vi "MeasureFastIV.vi"(0 ".NET Refnum in":refnum<k24>, 1 ".NET Refnum":refnum<k24>, 2 "Junction Name":string, 7 "appended path":path, 12 "new file path (Not A Path if cancelled)":path, 13 "UiDefinition":T1, 14 "Function":string) -> (15 "error out":errorcluster)   [LabVIEW 2020]
uses:
  D:/LabviewDXFViewer/LabviewDXFViewer/bin/Release/LabviewDXFViewer.exe
  LabviewDXFViewer/bin/Release/LabviewDXFViewer.exe
  UIReferences.ctl
  <vilib>/Analysis/6fits.llb/Curve Fitting Criteria.ctl
  <vilib>/Utility/file.llb/Write Delimited Spreadsheet (DBL).vi
  <vilib>/Utility/file.llb/Write Delimited Spreadsheet (string).vi
  <vilib>/Analysis/NI_AALPro.lvlib
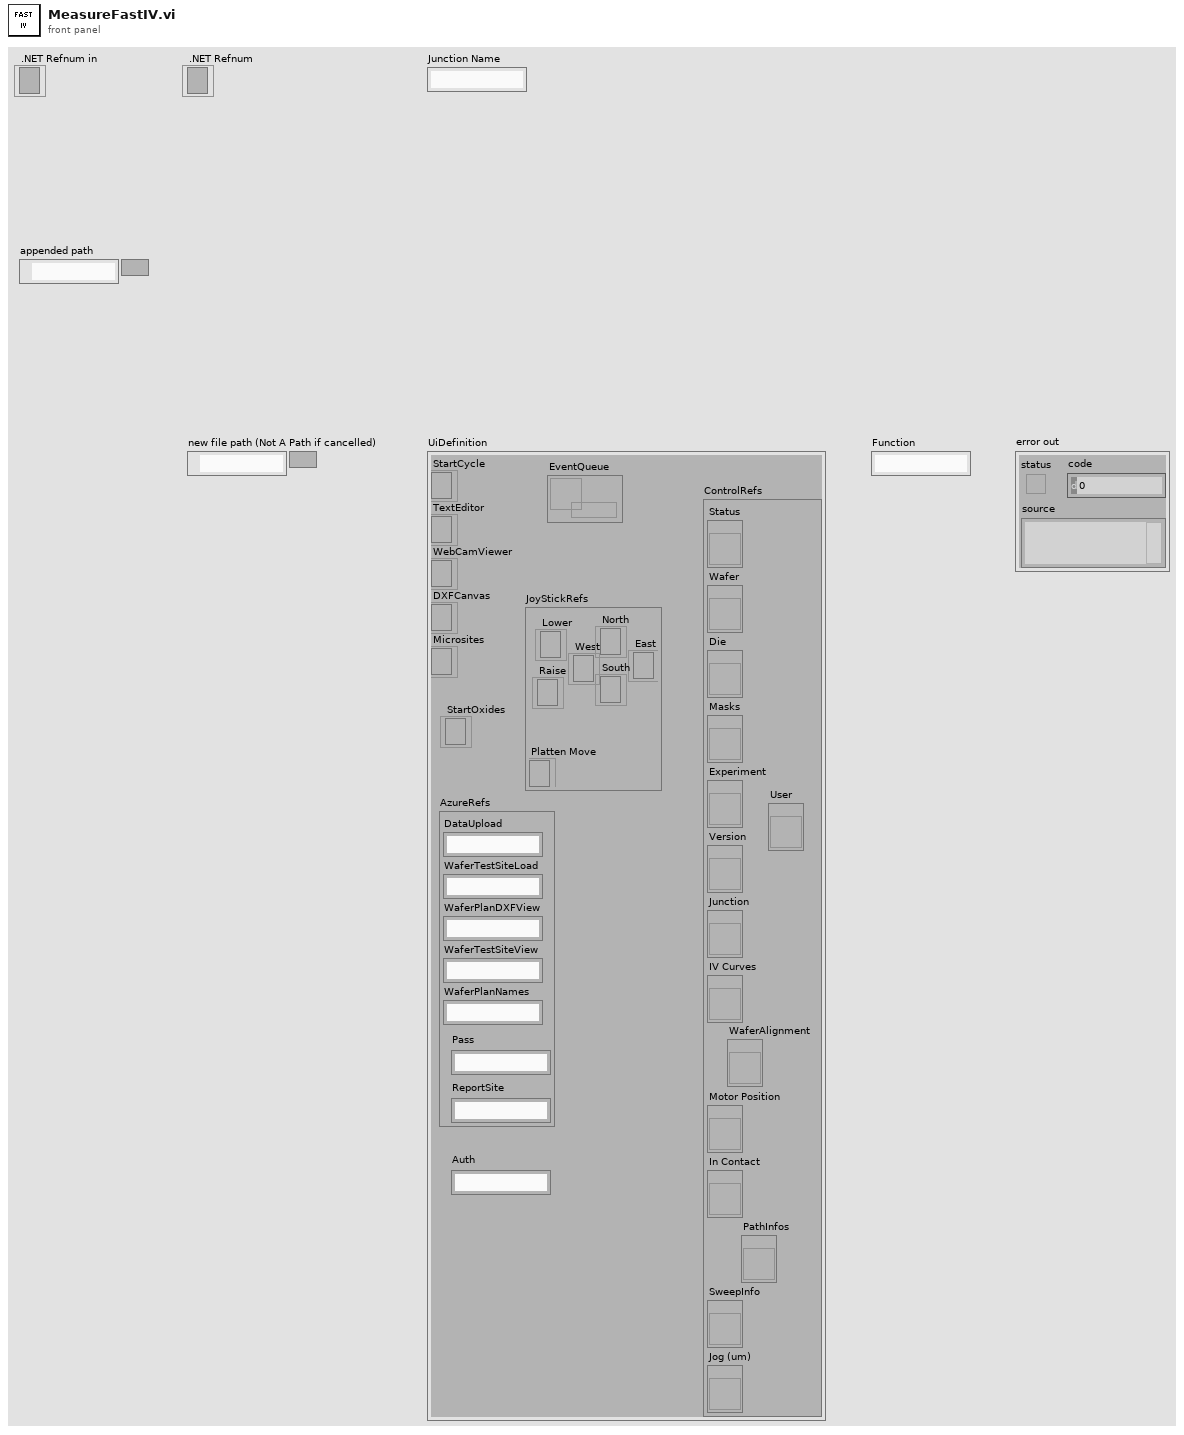
[diagram p1: front panel]
types:
  T1 = typedef "UIReferences.ctl" = cluster{"StartCycle":refnum<k24>, "TextEditor":refnum<k24>, "WebCamViewer":refnum<k24>, "DXFCanvas":refnum<k24>, "Microsites":refnum<k24>, "JoyStickRefs":cluster{"North":refnum<k24>, "Lower":refnum<k24>, "Raise":refnum<k24>, "Platten Move":refnum<k24>, "West":refnum<k24>, "East":refnum<k24>, "South":refnum<k24>}, "AzureRefs":cluster{"DataUpload":string, "WaferTestSiteLoad":string, "WaferPlanDXFView":string, "WaferTestSiteView":string, "WaferPlanNames":string, "Pass":string, "ReportSite":string}, "ControlRefs":cluster{"Status":refnum<vi>, "Wafer":refnum<vi>, "Die":refnum<vi>, "Masks":refnum<vi>, "Experiment":refnum<vi>, "Version":refnum<vi>, "Junction":refnum<vi>, "IV Curves":refnum<vi>, "Motor Position":refnum<vi>, "In Contact":refnum<vi>, "SweepInfo":refnum<vi>, "Jog (um)":refnum<vi>, "PathInfos":refnum<vi>, "User":refnum<vi>, "WaferAlignment":refnum<vi>}, "EventQueue":refnum<queue>, "StartOxides":refnum<k24>, "Auth":string}
  T2 = typedef "NI_AALPro.lvlib/Curve Fitting Criteria.ctl" = u16
  T3 = cluster{"Current Range":dbl, "Source Measure Unit Channel (0: Channel A)":i32, "Waveform":waveform(dbl), "VISA resource name":refnum<visa-resource-name>, "CodeText":string}
  T4 = typedef "CapacitanceInfos.ctl" = cluster{"Conductance":dbl, "CapacitanceIV":dbl, "Intercept":dbl, "CapacitanceSW":dbl, "Sum":dbl, "CapacitanceInfos":T5[], "CapacitancePhase":dbl, "dC/dV":dbl, "Function":string, "OtherInfo":dbl[][]}
  T5 = typedef "CapacitanceRecord.ctl" = cluster{"Freq":dbl, "Vpp":dbl, "PhaseS":dbl, "Irms":dbl, "PhaseC":dbl, "Theta":dbl, "VDrive":dbl, "Capacitance":dbl, "Other":dbl}
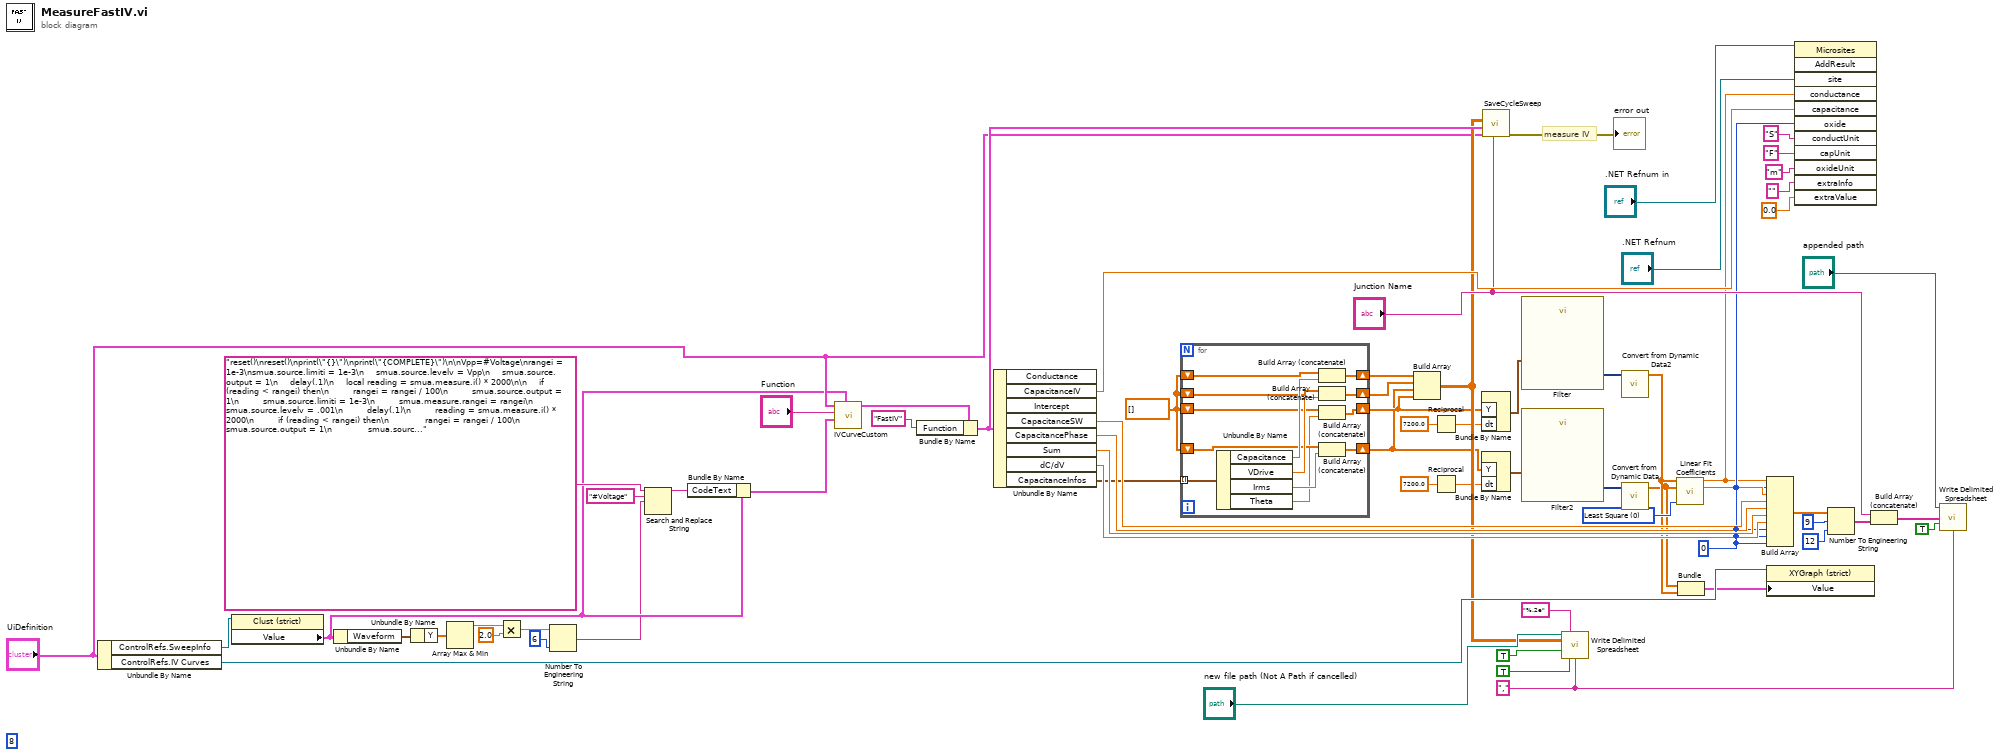
[diagram p0: block diagram]
diagram:
  w9 = 0
  (unwired) i16 8 ("width (-)")
  w32 = T2 0 items=["Least Square", "Least Absolute Residual", "Bisquare"] ("method")
  w36 = dbl[] []
  w44 = "," ("delimiter (\\t)")
  # "measure IV"
  n1 = Unbundle By Name("UiDefinition") -> ("ControlRefs.SweepInfo"=w42:refnum<vi>, "ControlRefs.IV Curves"=w38:refnum<vi>)
  n2 = property class="Clust (strict)"(reference=w42) -> ("Value"=w18:T3)  [unwired: 1 in, 2 out]
  n3 = Unbundle By Name(w18) -> ("Waveform"=w27:waveform(dbl))
  n4 = Unbundle By Name(w27) -> ("Y"=w26:dbl[])
  n5 = Array Max & Min(array=w26) -> (max value=w25:dbl)  [unwired: 3 out]
  n6 = Multiply(x=w25, y=2.0) -> (x*y=w17:dbl)
  n7 = Number To Engineering String(2:i16 6 ("precision (6)"), 4:w17) -> (0:w15:string)  [unwired: 2 in]
  n8 = Search and Replace String(input string="reset()\nreset()\nprint(\"{}\")\nprint(\"{COMPLETE}\")\n\nVpp=#Voltage\nrangei = 1e-3\nsmua.source.limiti = 1e-3\n    smua.source.levelv = Vpp\n    smua.source.output = 1\n    delay(.1)\n    local reading = smua.measure.i() * 2000\n\n    if (reading < rangei) then\n        rangei = rangei / 100\n        smua.source.output = 1\n        smua.source.limiti = 1e-3\n        smua.measure.rangei = rangei\n        smua.source.levelv = .001\n        delay(.1)\n        reading = smua.measure.i() * 2000\n        if (reading < rangei) then\n            rangei = rangei / 100\n            smua.source.output = 1\n            smua.source.limiti = 1e-3\n            smua.measure.rangei = rangei\n            smua.source.levelv = .001\n            delay(.1)\n            reading = smua.measure.i() * 2000\n            if (reading < rangei) then\n                rangei = rangei / 1000\n                doCap =1\n                smua.source.levelv = 0\n            end\n        end\n    end\n\n\nVLin=0\nnumCycles=5\nfrequency=10\nlimitI=rangei\nskips=0\ndisplay=1\n\nreset()\n\tlocal COMPLETE = \"{COMPLETE}\"\n\t-- Generate the source values\n\n\tlocal sourceValues\t\t= {} \n\tlocal pointsPerCycle\t= 7200 / frequency\n\tlocal numDataPoints\t\t= pointsPerCycle * numCycles\n\n\np=pointsPerCycle/2\nlocal x=p/2.0\n    for i = 1, numDataPoints do\n\t    c=math.mod(x,2*p)\n\n        y = Vpp/p*(math.abs(c-p ));\n\n        sourceValues[i] =y-Vpp/2\n\nx=x+1\n    end\n\n\t-- Configure the SMU ranges\n\tsmua.reset()\n\tsmua.source.settling\t\t= smua.SETTLE_FAST_POLARITY\n\tsmua.source.autorangev\t\t= smua.AUTORANGE_OFF\n\tsmua.source.autorangei\t\t= smua.AUTORANGE_OFF\n    smua.source.rangev\t\t\t= 1\n\tsmua.source.delay\t\t\t= 0\n\tsmua.source.limiti\t\t\t= limitI\n\n\tsmua.measure.autorangev\t\t= smua.AUTORANGE_OFF\n\tsmua.measure.autorangei\t\t= smua.AUTORANGE_OFF\n\tsmua.measure.autozero\t\t= smua.AUTOZERO_OFF\n\tsmua.measure.delay\t\t\t= 0\n\tsmua.measure.delayfactor    = 1\n\tsmua.measure.analogfilter   = 0\n\n\t-- Voltage will be measured on the same range as the source range\n\tsmua.measure.rangei\t\t\t= limitI\n\tsmua.measure.nplc\t\t\t= 0.001\n\n\t-- Prepare the Reading Buffers\n\tsmua.nvbuffer1.clear()\n\tsmua.nvbuffer1.collecttimestamps\t= 1\n\tsmua.nvbuffer2.clear()\n\tsmua.nvbuffer2.collecttimestamps\t= 1\n\n\t-- Configure the trigger model\n\t--============================\n\t\n\t-- Timer 1 controls the time between source points\n\ttrigger.timer[1].delay = (1 / 7200)\n\ttrigger.timer[1].passthrough = true\n\ttrigger.timer[1].stimulus = smua.trigger.ARMED_EVENT_ID\n\ttrigger.timer[1].count = numDataPoints - 1\n\n\t-- Configure the SMU trigger model\n\tsmua.trigger.source.listv(sourceValues)\n\tsmua.trigger.source.limiti\t\t= limitI\n\tsmua.trigger.measure.action\t\t= smua.ENABLE\n\tsmua.trigger.measure.iv(smua.nvbuffer1, smua.nvbuffer2)\n\tsmua.trigger.endpulse.action\t= smua.SOURCE_HOLD\n\tsmua.trigger.endsweep.action\t= smua.SOURCE_IDLE\n\tsmua.trigger.count\t\t\t\t= numDataPoints\n\tsmua.trigger.arm.stimulus\t\t= 0\n\tsmua.trigger.source.stimulus\t= trigger.timer[1].EVENT_ID\n\tsmua.trigger.measure.stimulus\t= 0\n\tsmua.trigger.endpulse.stimulus\t= 0\n\tsmua.trigger.source.action\t\t= smua.ENABLE\n\t-- Ready to begin the test\n\n\tsmua.source.output\t\t\t\t\t= smua.OUTPUT_ON\n\t-- Start the trigger model execution\n\tsmua.trigger.initiate()\n\t-- Wait until the sweep has completed\n\twaitcomplete()\n\tsmua.source.output\t\t\t\t\t= smua.OUTPUT_OFF\n\n\t-- Print the data back to the Console in tabular format\n\n    for x=pointsPerCycle, smua.nvbuffer2.n do\n\n     readingV=smua.nvbuffer2[x]\n     readingI=smua.nvbuffer1[x]\n\n      \n            print(0, 1, 0,smua.nvbuffer1.timestamps[x] ,0 , 0, 0,readingV,readingI)\n\n\nend\n\nprint(\"{COMPLETE}\")\n\n        smua.source.output = smua.OUTPUT_OFF" ("CodeText"), search string="#Voltage", replace string=w15) -> (result string=w23:string)  [unwired: 5 in, 3 out]
  n9 = Bundle By Name(cluster=w18, "CodeText"=w23) -> (w22:T3)
  n10 = call "IVCurveCustom.vi"("OriginalSweepInfo"=w18, "SweepInfo"=w22, "Program"="Function", "UiDefinition"="UiDefinition") -> ("InfoCluster"=w19:T4)  [unwired: 6 in, 1 out]
  n11 = Bundle By Name(cluster=w19, "Function"="FastIV") -> (w41:T4)
  n12 = Unbundle By Name(w41) -> ("CapacitanceIV"=w67:dbl, "CapacitanceSW"=w59:dbl, "CapacitancePhase"=w60:dbl, "Sum"=w57:dbl, "dC/dV"=w58:dbl, "CapacitanceInfos"=w37:T5[])  [unwired: 2 out]
  n13 = for {
    tunnel: w37 -> [w79] mode=indexing
    shift-right: [w80] -> w33
    shift-left: w36 -> [w77]
    shift-right: [w76] -> w35
    shift-left: w36 -> [w75]
    shift-right: [w72] -> w2
    shift-left: w36 -> [w73]
    shift-right: [w70] -> w7
    shift-left: w36 -> [w71]
    n14 = Unbundle By Name(w79) -> ("Capacitance"=w78:dbl, "VDrive"=w74:dbl, "Irms"=w69:dbl, "Theta"=w68:dbl)
    n15 = Build Array (concatenate)(w77, w78) -> (w80:dbl[])
    n16 = Build Array (concatenate)(w75, w74) -> (w76:dbl[])
    n17 = Build Array (concatenate)(w71, w68) -> (w70:dbl[])
    n18 = Build Array (concatenate)(w73, w69) -> (w72:dbl[])
  }
  n19 = Build Array(w33, w35, w2, w7) -> (w34:dbl[][])
  n20 = Reciprocal(x=7200.0 ("dt")) -> (1/x=w12:dbl)
  n21 = Reciprocal(x=7200.0 ("dt")) -> (1/x=w4:dbl)
  n22 = Bundle By Name("Y"=w7, "dt"=w12) -> (w11:waveform(dbl))  [unwired: 1 in]
  n23 = Bundle By Name("Y"=w2, "dt"=w4) -> (w3:waveform(dbl))  [unwired: 1 in]
  n24 = call "SaveCycleSweep.vi"("JunctionName"="Junction Name", "UiDefinition 2"="UiDefinition", "InfoCluster"=w41, "appended array"=w34) -> ("error out"=→"error out":errorcluster)  [unwired: 7 in]
  n25 = call "Filter"("Signal"=w11) -> ("Filtered Signal"=w14:dynamicdata)  [unwired: 9 in, 1 out]
  n26 = call "Filter2"("Signal"=w3) -> ("Filtered Signal"=w6:dynamicdata)  [unwired: 9 in, 1 out]
  n27 = call-poly <vilib>:"Write Delimited Spreadsheet.vi"("file path (dialog if empty)"="new file path (Not A Path if cancelled)", "format (%.3f)"="%.2e", "2D data"=w34, "append to file? (new file:F)"=TRUE, "transpose? (no:F)"=TRUE, "delimiter (\\t)"=w44) -> ()  [unwired: 8 in, 2 out]
  n28 = call "Convert from Dynamic Data2"("Dynamic Data Type"=w14) -> ("Array"=w10:dbl[])  [unwired: 3 in]
  n29 = call "Convert from Dynamic Data"("Dynamic Data Type"=w6) -> ("Array"=w1:dbl[])  [unwired: 3 in]
  n30 = call <vilib>:"Linear Fit Coefficients.vi"("Y"=w10, "X"=w1, "method"=w32) -> ("slope"=w8:dbl, "intercept"=w31:dbl)  [unwired: 10 in, 1 out]
  n31 = Bundle("Array"=w1, "Array"=w10) -> (w30:cluster{"Array":dbl[], "Array":dbl[]})  [unwired: 1 in]
  n32 = Build Array(w8, w9, w31, w59, w60, w57, w58, w9, w9, w9) -> (w56:dbl[])
  n33 = property class="XYGraph (strict)"(reference=w38, "Value"=w30) -> ()  [unwired: 1 in, 2 out]
  n34 = invoke class="Microsites" method="AddResult"(reference=".NET Refnum in", "site"=".NET Refnum", "conductance"=w8, "capacitance"=w67, "oxide"=w9, "conductUnit"="S", "capUnit"="F", "oxideUnit"="m" ("interceptUnit"), "extraInfo"="", "extraValue"=0.0) -> ()  [unwired: 2 in, 12 out]
  n35 = Number To Engineering String(2:i16 12 ("precision (6)"), 3:i16 9 ("width (-)"), 4:w56) -> (0:w49:string[])  [unwired: 1 in]
  n36 = Build Array (concatenate)("Junction Name", w49) -> (w51:string[])
  n37 = call-poly <vilib>:"Write Delimited Spreadsheet.vi"("file path (dialog if empty)"="appended path", "1D data"=w51, "append to file? (new file:F)"=TRUE, "delimiter (\\t)"=w44) -> ()  [unwired: 10 in, 2 out]
